vi "DCPower_Reconfig_byInstrument_perChannel.vi"(2 "error in (no error)":errorcluster, 3 "DCPower_byInstrument_input":T1(array[cluster])) -> (0 "error out":errorcluster, 1 "DCPowerInformation_byInstrument":T1(array[cluster]))   [LabVIEW 2019]
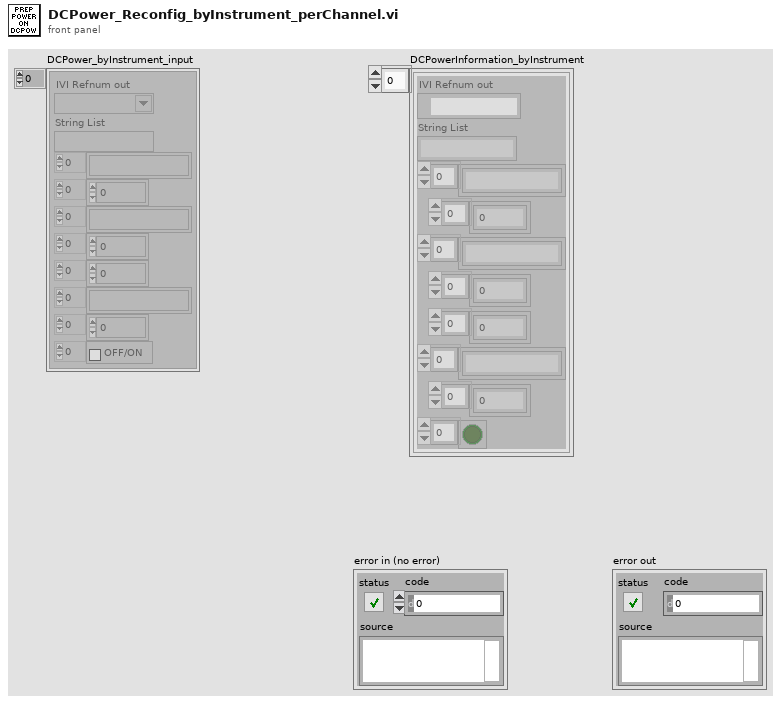
[diagram p1: front panel]
types:
  T1 = cluster{"IVI Refnum out":refnum<k15>, "String List":string, string[], dbl[], string[], dbl[], dbl[], string[], dbl[], bool[]}[]
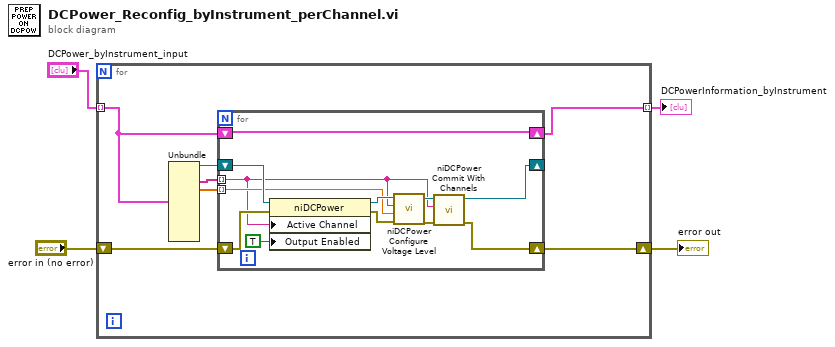
[diagram p0: block diagram]
diagram:
  n1 = for {
    shift-right: [w8] -> w3
    shift-left: "error in (no error)" -> [w9]
    tunnel: "DCPower_byInstrument_input" -> [w6] mode=indexing
    tunnel: [w7] -> w1 mode=indexing
    n2 = Unbundle(w6) -> ("IVI Refnum out"=w5:refnum<k15>, w10:string[], w11:dbl[])  [unwired: 7 out]
    n3 = for {
      shift-right: [w13] -> _
      shift-left: w5 -> [w16]
      shift-right: [w21] -> w7
      shift-left: w6 -> [w21]
      shift-right: [w12] -> w8
      shift-left: w9 -> [w17]
      tunnel: w10 -> [w14] mode=indexing
      tunnel: w11 -> [w15] mode=indexing
      n4 = property class="niDCPower"(reference=w16, error in=w17, "Active Channel"=w14, "Output Enabled"=TRUE ("Source:Output Enabled")) -> (reference out=w18:refnum<k15>, error out=w19:errorcluster)
      n5 = call <instrlib>:"niDCPower Configure Voltage Level.vi"("error in (no error)"=w19, "voltage level"=w15, "channel name"=w14, "instrument handle"=w18) -> ("error out"=w23:errorcluster, "instrument handle out"=w22:refnum<k15>)  [unwired: 6 in]
      n6 = call <instrlib>:"niDCPower Commit With Channels.vi"("error in (no error)"=w23, "channel name"=w14, "instrument handle"=w22) -> ("error out"=w12:errorcluster, "instrument handle out"=w13:refnum<k15>)  [unwired: 7 in]
    }
  }
  "error out" <- w3
  "DCPowerInformation_byInstrument" <- w1
